vi "RP Read Status TCP.vi"(4 "bytes to read":i32=4, 6 "timeout ms (25000)":i32=1000, 8 "Error In":errorcluster, 9 "Status offset":u64, 10 "Read config":bool, 11 "connection ID":refnum<k5>) -> (0 "Error Out":errorcluster, 1 "Status response":u32=1 format="0x%x (%d)", 3 "connection ID out":refnum<k5>)   [LabVIEW 2024]
uses:
  RP Command.ctl
panel:
  out "bytes written":i32
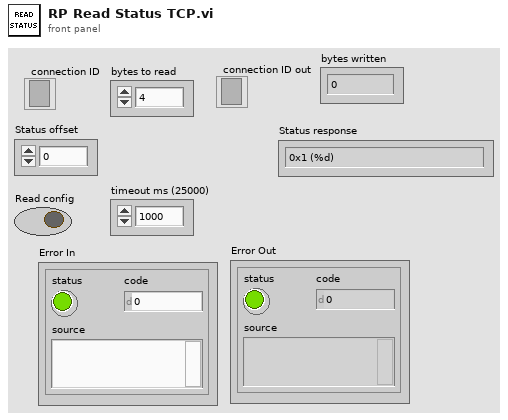
[diagram p1: front panel]
types:
  T1 = typedef "RP Command.ctl" = enum16{"Reset", "Read IDN", "Stop server", "Get status", "Get temperature", "Connect client", "Arm", "Software trigger", "Get whole buffer", "Get chunk", "System call", "Get config", "Set config", "Recieve data", "Recieve Calibartion", "Transmit data"}
  T2 = enum16{"big-endian, network order", "native, host order", "little-endian"}
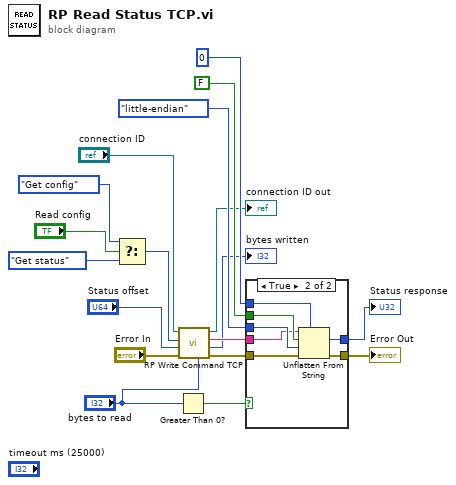
[diagram p0: block diagram]
diagram:
  n1 = Select(t=RP_Command."Get config" ("Command number"), s="Read config", f=RP_Command."Get status" ("Command number")) -> (s? t:f=w5:T1)
  n2 = Greater Than 0?(x="bytes to read") -> (x > 0?=w1:bool)
  n3 = call "RP Write Command TCP.vi"("bytes to read"="bytes to read", "Error In"="Error In", "Command payload"="Status offset", "Command number"=w5, "connection ID"="connection ID") -> ("Error Out"=w14:errorcluster, "bytes written"=→"bytes written":i32, "data out"=w4:string, "connection ID out"=→"connection ID out":refnum<k5>)  [unwired: 3 in]
  n4 = case shown="True" w1 {
    tunnel: FALSE ("data includes array or string size? (T)") -> [_ w26]
    tunnel: w14 -> [w19 w25]
    tunnel: u32 0 -> [_ w24]
    tunnel: T2."little-endian" ("byte order (0:big-endian, network order)") -> [_ w23]
    tunnel: [_ w22] -> w11
    tunnel: [w19 w21] -> w10
    tunnel: w4 -> [_ w20]
    frame False {
    }
    frame True {
      n5 = Unflatten From String(type=w24, binary string=w20, data includes array or string size? (T)=w26, byte order (0:big-endian, network order)=w23, error in (no error)=w25) -> (value=w22:u32, error out=w21:errorcluster)  [unwired: 1 out]
    }
  }
  "Error Out" <- w10
  "Status response" <- w11
